vi "TunnelMode(ForLoop).vi"() -> ()   [LabVIEW 2023]
panel:
  out "number: 0 to 1":dbl
  out "Array":dbl[](array[numeric])
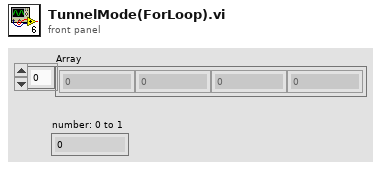
[diagram p1: front panel]
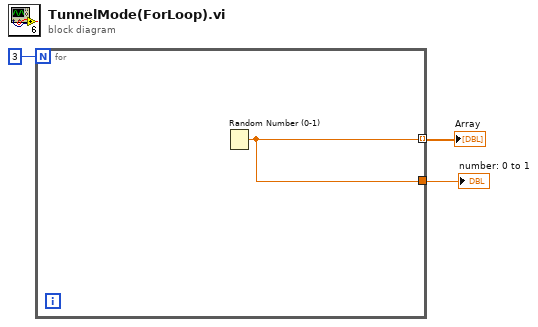
[diagram p0: block diagram]
diagram:
  n1 = for {
    N: 3 -> [_]
    tunnel: [w4] -> w2 mode=indexing
    tunnel: [w4] -> w1
    n2 = Random Number (0-1)() -> (number: 0 to 1=w4:dbl)
  }
  "Array" <- w2
  "number: 0 to 1" <- w1
